vi "2D Array Comparison.vi"() -> ()   [LabVIEW 2013]
panel:
  out "Masked Array":i32[][](array[numeric])
  in  "Processing Times":u16[][](array[numeric])=[[34, 15, 38, 95], [2, 89, 19, 7], [54, 70, 28, 34], [61, 9, 87, 29]]
  out "Remaining Processing Times":u16[][](array[numeric])
  out "x = y?":bool[][](array[boolean])
  out "Indices of Identical Elements":i32[][](array[numeric])
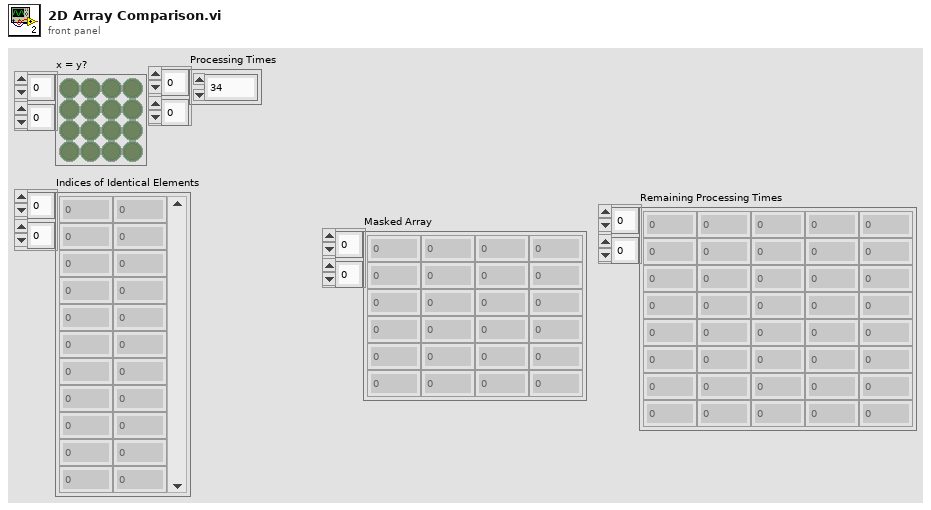
[diagram p1: front panel]
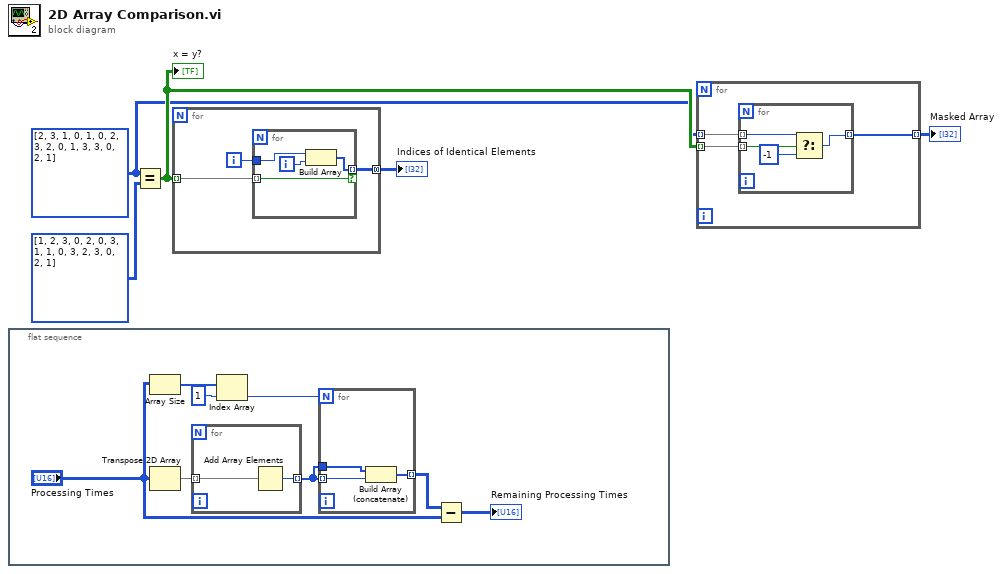
[diagram p0: block diagram]
diagram:
  w2 = i32[][] [[2, 3, 1, 0], [1, 0, 2, 3], [2, 0, 1, 3], [3, 0, 2, 1]] ("Job Schedule on Machine")
  n1 = flat-sequence {
    frame #0 {
      n2 = Array Size(array="Processing Times") -> (size(s)=w12:i32[])
      n3 = Transpose 2D Array(2D array="Processing Times") -> (transposed array=w13:u16[][])
      n4 = for {
        tunnel: w13 -> [w18] mode=indexing
        tunnel: [w17] -> w9 mode=indexing
        n5 = Add Array Elements(numeric array=w18) -> (sum=w17:u16)
      }
      n6 = Index Array(array=w12, index=1) -> (element=w11:i32)
      n7 = for {
        N: w11 -> [_]
        tunnel: w9 -> [w15] mode=indexing
        tunnel: w9 -> [w16]
        tunnel: [w14] -> w8 mode=indexing
        n8 = Build Array (concatenate)(w16, w15) -> (w14:u16[])
      }
      n9 = Subtract(x=w8, y="Processing Times") -> (x-y=→"Remaining Processing Times":u16[][])
    }
  }
  n10 = Equal?(x=w2, y=i32[][] [[1, 2, 3, 0], [2, 0, 3, 1], [1, 0, 3, 2], [3, 0, 2, 1]] ("Job Schedule on Machine")) -> (x = y?=w3:bool[][])
  "x = y?" <- w3
  n11 = for {
    tunnel: w3 -> [w21] mode=indexing
    tunnel: [w20] -> w4 mode=concatenating
    i -> [w19]
    n12 = for {
      tunnel: w21 -> [w25] mode=indexing
      tunnel: [w23] -> w20 mode=indexing if=w25
      tunnel: w19 -> [w22]
      i -> [w24]
      n13 = Build Array(w22, w24) -> (w23:i32[])
    }
  }
  "Indices of Identical Elements" <- w4
  n14 = for {
    tunnel: w3 -> [w27] mode=indexing
    tunnel: w2 -> [w28] mode=indexing
    tunnel: [w26] -> w1 mode=indexing
    n15 = for {
      tunnel: w28 -> [w31] mode=indexing
      tunnel: w27 -> [w32] mode=indexing
      tunnel: [w29] -> w26 mode=indexing
      n16 = Select(t=w31, s=w32, f=-1) -> (s? t:f=w29:i32)
    }
  }
  "Masked Array" <- w1
